vi "Zero Distance.vi"(8 "error in (no error)":errorcluster, 11 "Motors with Encoders in":refnum<class "Motors with Encoders.lvclass">) -> (0 "error out":errorcluster, 3 "Motors with Encoders out":refnum<class "Motors with Encoders.lvclass">)   [LabVIEW 2014, in "Motors with Encoders.lvlib" / "Motors with Encoders.lvclass"]
uses:
  Motors with Encoders.lvclass
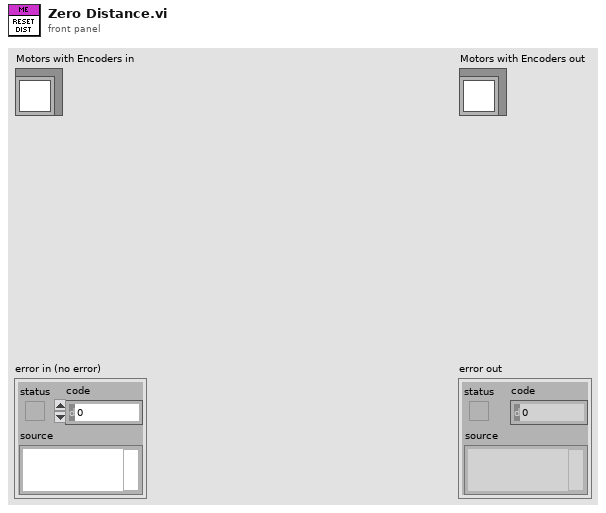
[diagram p1: front panel]
types:
  T1 = typedef "Motors with Encoders.lvlib/Motors with Encoders.lvclass/Motors with Encoders State.ctl" = cluster{"Forward Switch":bool, "Reverse Switch":bool, "Measured RPM":dbl, "Distance (in)":dbl, "Setpoint RPM":dbl, "Encoder Count":i64, "Home Count":i64, "Config":T2}
  T2 = typedef "Motors with Encoders.lvlib/Motors with Encoders.lvclass/Motors with Encoders Config.ctl" = cluster{"Counts  Per Revolution":u32, "Invert Encoder Direction":bool, "Diameter of Revolution":dbl, "Max RPM":dbl, "Encoder Control":bool}
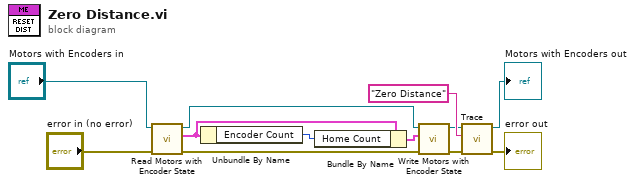
[diagram p0: block diagram]
diagram:
  n1 = call-dynamic "Read Motors with Encoder State.vi"("error in (no error)"="error in (no error)", "Motors with Encoders in"="Motors with Encoders in") -> ("error out"=w9:errorcluster, "Motors with Encoder State"=w2:T1, "Motors with Encoders out"=w8:refnum<class "Motors with Encoders.lvclass">)  [unwired: 7 in]
  n2 = Unbundle By Name(w2) -> ("Encoder Count"=w1:i64)
  n3 = Bundle By Name(cluster=w2, "Home Count"=w1) -> (w6:T1)
  n4 = call-dynamic "Write Motors with Encoder State.vi"("error in (no error)"=w9, "Motors with Encoder State"=w6, "Motors with Encoders in"=w8) -> ("error out"=w3:errorcluster, "Motors with Encoders out"=w5:refnum<class "Motors with Encoders.lvclass">)  [unwired: 7 in]
  n5 = call-dynamic "Trace.vi"("error in (no error)"=w3, "System Action"="Zero Distance", "System Actor in"=w5) -> ("error out"=→"error out":errorcluster, "System Actor out"=→"Motors with Encoders out":refnum<class "Motors with Encoders.lvclass">)  [unwired: 7 in]
